vi "nanomsg_new_event.vi"(3 "error in":errorcluster, 5 "event ref in (new event)":refnum<event-registration>) -> (0 "error out":errorcluster, 1 "user event":refnum<user-event>, 2 "event ref out":refnum<event-registration>)   [LabVIEW 2014, in "nanomsg.lvlib" / "nanomsg_socket.lvclass"]
doc: "Registers an event handler for a Nanomsg polling event, which can be fed into an Event Structure to trigger an event on message received using nn_recv/nn_recvmsg"
uses:
  nanomsg_socket.lvclass
  poll_event_data.ctl
  nanomsg.lvlib
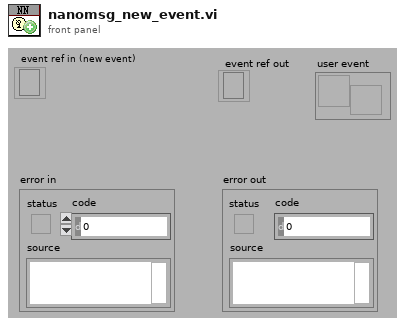
[diagram p1: front panel]
types:
  T1 = typedef "nanomsg.lvlib/poll_event_data.ctl" = cluster{"identity":string, "data":string[]}
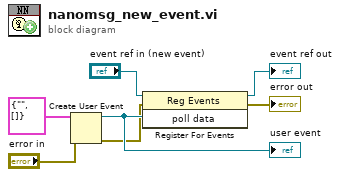
[diagram p0: block diagram]
diagram:
  n1 = Create User Event(user event datatype=T1 {"identity"="", "data"=[]} ("poll data"), error in="error in") -> (user event=w6:refnum<user-event>, error out=w3:errorcluster)
  "user event" <- w6
  n2 = register-events(reference="event ref in (new event)", error in=w3, w6) -> (reference out=→"event ref out":refnum<event-registration>, error out=→"error out":errorcluster)
